vi "GetDataSourceItem.vi"(10 "data source id":string, 11 "DataSourceItems in":variant) -> (1 "found":bool, 2 "DataSourceItem":T1, 3 "DataSourceItems out":variant)   [LabVIEW 2017, in "DeviceModelHelpers.lvlib"]
uses:
  <vilib>/addons/InsightCM/Utilities/DeviceModelHelpers/DeviceModelHelpers.lvlib
  <vilib>/addons/InsightCM/MessageBus/Base/controls/DataSourceItem.ctl
  <vilib>/addons/InsightCM/MessageBus/Base/controls/KeyValuePair.ctl
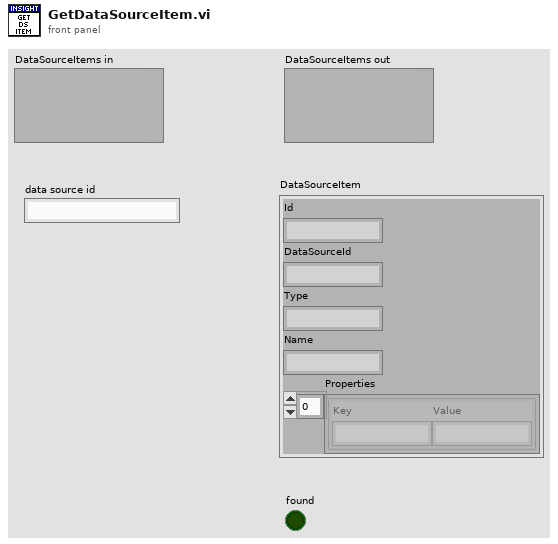
[diagram p1: front panel]
types:
  T1 = typedef "DataSourceItem.ctl" = cluster{"Id":string, "DataSourceId":string, "Type":string, "Name":string, "Properties":T2[]}
  T2 = typedef "KeyValuePair.ctl" = cluster{"Key":string, "Value":string}
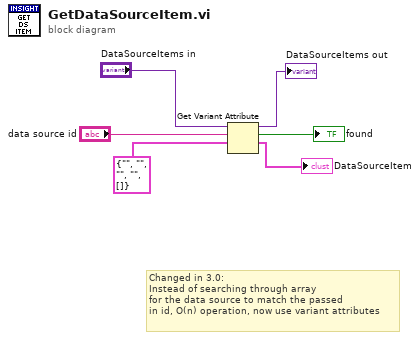
[diagram p0: block diagram]
diagram:
  # "Changed in 3.0:\nInstead of searching through array\nfor the data source to match the passed\nin id, O(n) operation, now use variant attributes"
  n1 = Get Variant Attribute(Variant="DataSourceItems in", name="data source id", default value (empty Variant)=T1 {"Id"="", "DataSourceId"="", "Type"="", "Name"="", "Properties"=[]} ("DataSourceItem")) -> (duplicate Variant=→"DataSourceItems out":variant, found=→"found":bool, value=→"DataSourceItem":T1)  [unwired: 1 in, 1 out]
